vi "Testing.vi"() -> ()   [LabVIEW 2023]
uses:
  Communication/PCAN2023/PCAN API.lvlib
panel:
  out "Read NTCs 2":bool
  out "Set Vehicle Speed 2":bool
  out "Read System Status 2":bool
  out "Connect2 2":bool
  out "Clear Nexteer NTCs 2":bool
  out "Enable Engine Run 2":bool
  out "Read MEC Counter 2":bool
  out "Write Polarity 2":bool
  out "Write BEMF 2":bool
  out "Write System Friction 2":bool
  out "Write Analog Torque Scale 7":bool
  out "Write Analog Torque Scale 6":bool
  out "Write Offset Values to default 2":bool
  out "Write Gain Values to default 2":bool
  out "Group 3":T1
  out "SW Version 4":bool
  out "SW Version 3":string
  out "Group1 2":T2
  out "Group1":T2
  out "SW Version 2":string
  out "SW Version":bool
  out "Nexteer Connect":bool
  out "error out":errorcluster
  in  "error in":errorcluster
  in  "Channel":u16=65 format="%x"
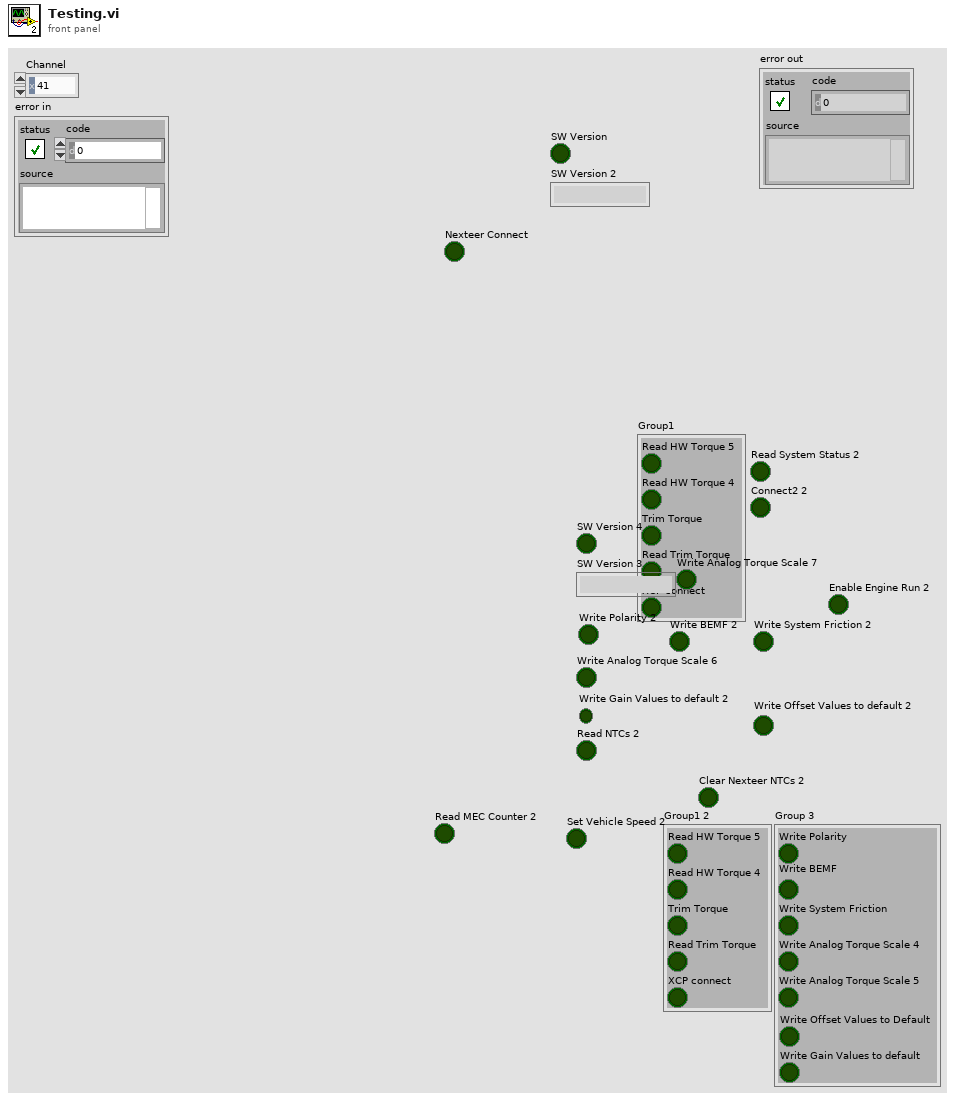
[diagram p1: front panel]
types:
  T1 = cluster{"Write Polarity":bool, "Write BEMF":bool, "Write System Friction":bool, "Write Analog Torque Scale 4":bool, "Write Analog Torque Scale 5":bool, "Write Gain Values to default":bool, "Write Offset Values to Default":bool}
  T2 = cluster{"Read HW Torque 5":bool, "Read HW Torque 4":bool, "Trim Torque":bool, "Read Trim Torque":bool, "XCP connect":bool}
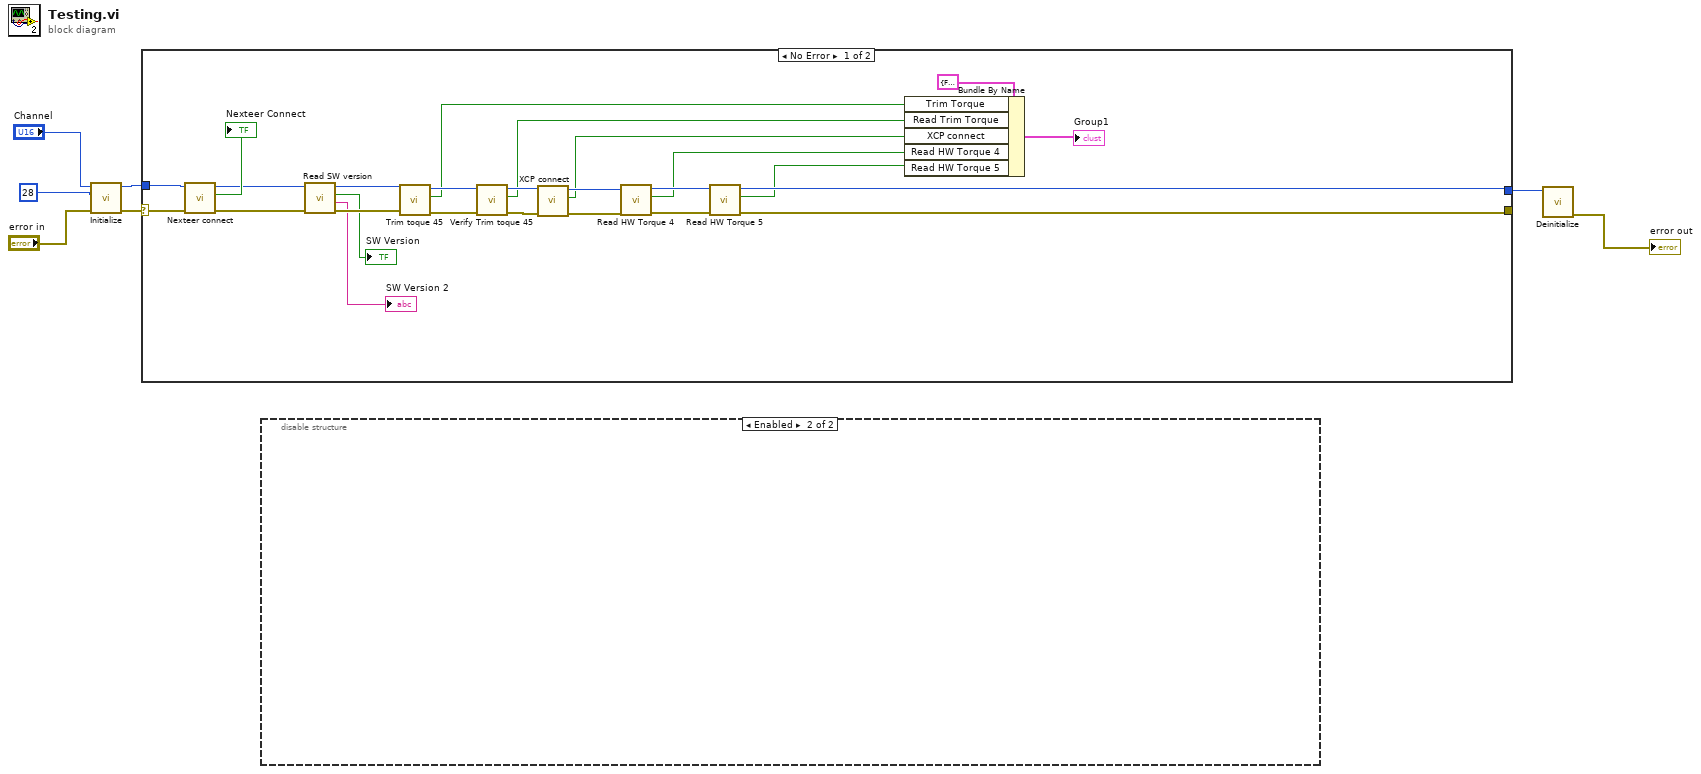
[diagram p0: block diagram]
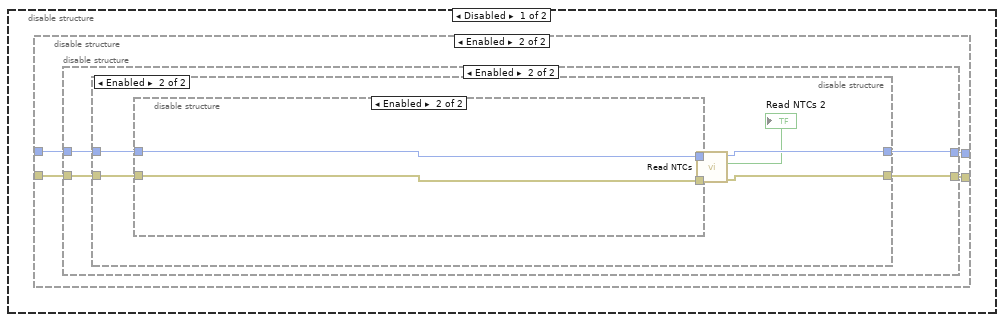
[diagram p2: hidden frame]
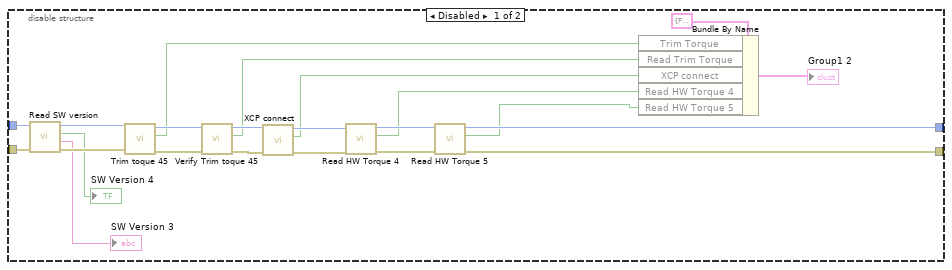
[diagram p3: hidden frame]
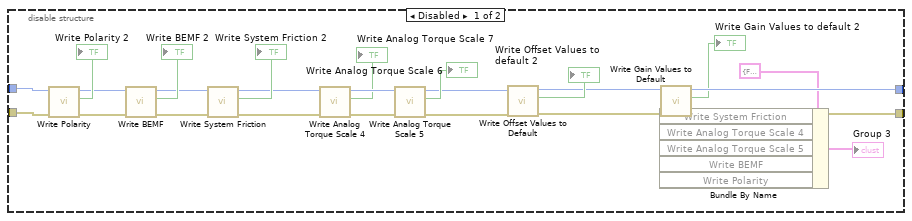
[diagram p4: hidden frame]
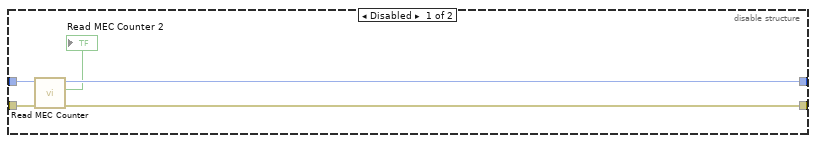
[diagram p5: hidden frame]
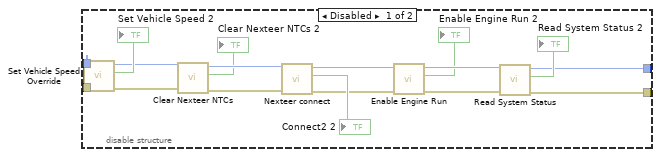
[diagram p6: hidden frame]
diagram:
  n1 = call "Initialize.vi"("error in"="error in", "Btr0Btr1"=u16 28, "Channel"="Channel") -> ("error out"=w1:errorcluster, "Channel out"=w4:u16)  [unwired: 6 in, 1 out]
  n2 = case shown="No Error" w1 {
    selector: w1 -> [w32 w35]
    tunnel: w4 -> [w33 w34]
    tunnel: [w28 w34] -> w3
    tunnel: [w27 w35] -> _
    frame No Error {
      n3 = call "Nexteer connect.vi"("error in"=w32, "Channel in"=w33) -> ("error out"=w29:errorcluster, "Pass"=→"Nexteer Connect":bool, "Channel out"=w30:u16)  [unwired: 4 in, 1 out]
      n4 = call "Read SW version.vi"("error in"=w29, "Channel in"=w30) -> ("error out"=w19:errorcluster, "SW Version"=→"SW Version 2":string, "Pass"=→"SW Version":bool, "Channel out"=w20:u16)  [unwired: 4 in]
      n5 = call "Trim toque 45.vi"("error in"=w19, "Channel in"=w20) -> ("error out"=w23:errorcluster, "Pass"=w12:bool, "Channel out"=w24:u16)  [unwired: 4 in, 1 out]
      n6 = call "Verify Trim toque 45.vi"("error in"=w23, "Channel in"=w24) -> ("error out"=w25:errorcluster, "Pass"=w11:bool, "Channel out"=w26:u16)  [unwired: 4 in, 1 out]
      n7 = call "XCP connect.vi"("error in"=w25, "Channel in"=w26) -> ("error out"=w21:errorcluster, "Pass"=w10:bool, "Channel out"=w22:u16)  [unwired: 4 in, 1 out]
      n8 = call "Read HW Torque 4.vi"("error in"=w21, "Channel in"=w22) -> ("error out"=w15:errorcluster, "Pass"=w9:bool, "Channel out"=w16:u16)  [unwired: 4 in, 1 out]
      n9 = call "Read HW Torque 5.vi"("error in"=w15, "Channel in"=w16) -> ("error out"=w27:errorcluster, "Pass"=w8:bool, "Channel out"=w28:u16)  [unwired: 4 in, 1 out]
      n10 = Bundle By Name(cluster=T2 {"Read HW Torque 5"=FALSE, "Read HW Torque 4"=FALSE, "Trim Torque"=FALSE, "Read Trim Torque"=FALSE, "XCP connect"=FALSE} ("Cluster 2"), "Trim Torque"=w12, "Read Trim Torque"=w11, "XCP connect"=w10, "Read HW Torque 4"=w9, "Read HW Torque 5"=w8) -> (→"Group1":T2)
    }
    frame Error {
    }
  }
  n11 = disable-structure shown="Enabled" {
    frame Disabled {
      n12 = disable-structure shown="Enabled" {
        disable-tunnel: _ -> [w52 w62]
        disable-tunnel: _ -> [w50 w61]
        disable-tunnel: [w45 w60] -> _
        disable-tunnel: [w43 w59] -> _
        frame Disabled {
          n13 = call "Read SW version.vi"("error in"=w50, "Channel in"=w52) -> ("error out"=w49:errorcluster, "SW Version"=→"SW Version 3":string, "Pass"=→"SW Version 4":bool, "Channel out"=w51:u16)  [unwired: 4 in]
          n14 = call "Trim toque 45.vi"("error in"=w49, "Channel in"=w51) -> ("error out"=w55:errorcluster, "Pass"=w40:bool, "Channel out"=w56:u16)  [unwired: 4 in, 1 out]
          n15 = call "Verify Trim toque 45.vi"("error in"=w55, "Channel in"=w56) -> ("error out"=w57:errorcluster, "Pass"=w39:bool, "Channel out"=w58:u16)  [unwired: 4 in, 1 out]
          n16 = call "XCP connect.vi"("error in"=w57, "Channel in"=w58) -> ("error out"=w53:errorcluster, "Pass"=w38:bool, "Channel out"=w54:u16)  [unwired: 4 in, 1 out]
          n17 = call "Read HW Torque 4.vi"("error in"=w53, "Channel in"=w54) -> ("error out"=w44:errorcluster, "Pass"=w37:bool, "Channel out"=w46:u16)  [unwired: 4 in, 1 out]
          n18 = call "Read HW Torque 5.vi"("error in"=w44, "Channel in"=w46) -> ("error out"=w43:errorcluster, "Pass"=w36:bool, "Channel out"=w45:u16)  [unwired: 4 in, 1 out]
          n19 = Bundle By Name(cluster=T2 {"Read HW Torque 5"=FALSE, "Read HW Torque 4"=FALSE, "Trim Torque"=FALSE, "Read Trim Torque"=FALSE, "XCP connect"=FALSE} ("Cluster 2"), "Trim Torque"=w40, "Read Trim Torque"=w39, "XCP connect"=w38, "Read HW Torque 4"=w37, "Read HW Torque 5"=w36) -> (→"Group1 2":T2)
        }
        frame Enabled {
          n20 = disable-structure shown="Enabled" {
            disable-tunnel: w62 -> [w88 w92]
            disable-tunnel: w61 -> [w87 w91]
            disable-tunnel: [w69 w90] -> w60
            disable-tunnel: [w67 w89] -> w59
            frame Disabled {
              n21 = call "Write Polarity.vi"("error in"=w87, "Channel in"=w88) -> ("error out"=w84:errorcluster, "Pass"=→"Write Polarity 2":bool, "Channel out"=w85:u16)  [unwired: 4 in, 1 out]
              n22 = call "Write BEMF.vi"("error in"=w84, "Channel in"=w85) -> ("error out"=w81:errorcluster, "Pass"=→"Write BEMF 2":bool, "Channel out"=w82:u16)  [unwired: 4 in, 1 out]
              n23 = call "Write System Friction.vi"("error in"=w81, "Channel in"=w82) -> ("error out"=w77:errorcluster, "Pass"=→"Write System Friction 2":bool, "Channel out"=w79:u16)  [unwired: 4 in, 1 out]
              n24 = call "Write Analog Torque Scale 4.vi"("error in"=w77, "Channel in"=w79) -> ("error out"=w76:errorcluster, "Pass"=→"Write Analog Torque Scale 7":bool, "Channel out"=w78:u16)  [unwired: 4 in, 1 out]
              n25 = call "Write Analog Torque Scale 5.vi"("error in"=w76, "Channel in"=w78) -> ("error out"=w72:errorcluster, "Pass"=→"Write Analog Torque Scale 6":bool, "Channel out"=w73:u16)  [unwired: 4 in, 1 out]
              n26 = call "Write Offset Values to Default.vi"("error in"=w72, "Channel in"=w73) -> ("error out"=w68:errorcluster, "Pass"=→"Write Offset Values to default 2":bool, "Channel out"=w70:u16)  [unwired: 4 in, 1 out]
              n27 = Bundle By Name(cluster=T1 {"Write Polarity"=FALSE, "Write BEMF"=FALSE, "Write System Friction"=FALSE, "Write Analog Torque Scale 4"=FALSE, "Write Analog Torque Scale 5"=FALSE, "Write Gain Values to default"=FALSE, "Write Offset Values to Default"=FALSE} ("Group 2")) -> (→"Group 3":T1, "Write Polarity"=w65:bool)  [unwired: 4 in]
              n28 = call "Write Gain Values to Default.vi"("error in"=w68, "Channel in"=w70) -> ("error out"=w67:errorcluster, "Pass"=→"Write Gain Values to default 2":bool, "Channel out"=w69:u16)  [unwired: 4 in, 1 out]
            }
            frame Enabled {
              n29 = disable-structure shown="Enabled" {
                disable-tunnel: w92 -> [w97 w104]
                disable-tunnel: w91 -> [w96 w103]
                disable-tunnel: [w95 w101] -> w90
                disable-tunnel: [w94 w99] -> w89
                frame Disabled {
                  n30 = call "Read MEC Counter.vi"("error in"=w96, "Channel in"=w97) -> ("error out"=w94:errorcluster, "Pass"=→"Read MEC Counter 2":bool, "Channel out"=w95:u16)  [unwired: 4 in, 1 out]
                }
                frame Enabled {
                  n31 = disable-structure shown="Enabled" {
                    disable-tunnel: w104 -> [w121 w123]
                    disable-tunnel: w103 -> [w120 w122]
                    disable-tunnel: [w106 w123] -> w102
                    disable-tunnel: [w105 w122] -> w100
                    frame Disabled {
                      n32 = call "Set Vehicle Speed Override.vi"("error in"=w120, "Channel in"=w121) -> ("error out"=w114:errorcluster, "Pass"=→"Set Vehicle Speed 2":bool, "Channel out"=w116:u16)  [unwired: 4 in, 1 out]
                      n33 = call "Clear Nexteer NTCs.vi"("error in"=w114, "Channel in"=w116) -> ("error out"=w113:errorcluster, "Pass"=→"Clear Nexteer NTCs 2":bool, "Channel out"=w115:u16)  [unwired: 4 in, 1 out]
                      n34 = call "Nexteer connect.vi"("error in"=w113, "Channel in"=w115) -> ("error out"=w109:errorcluster, "Pass"=→"Connect2 2":bool, "Channel out"=w111:u16)  [unwired: 4 in, 1 out]
                      n35 = call "Enable Engine Run.vi"("error in"=w109, "Channel in"=w111) -> ("error out"=w108:errorcluster, "Pass"=→"Enable Engine Run 2":bool, "Channel out"=w110:u16)  [unwired: 4 in, 1 out]
                      n36 = call "Read System Status.vi"("error in"=w108, "Channel in"=w110) -> ("error out"=w105:errorcluster, "Pass"=→"Read System Status 2":bool, "Channel out"=w106:u16)  [unwired: 4 in, 1 out]
                    }
                    frame Enabled {
                    }
                  }
                  n37 = call "Read NTCs.vi"("error in"=w100, "Channel in"=w102) -> ("error out"=w99:errorcluster, "Pass"=→"Read NTCs 2":bool, "Channel out"=w101:u16)  [unwired: 4 in, 1 out]
                }
              }
            }
          }
        }
      }
    }
    frame Enabled {
    }
  }
  n38 = call "Deinitialize.vi"("Channel"=w3) -> ("error out"=→"error out":errorcluster)  [unwired: 10 in]
